vi "Listbox demo.vi"() -> ()   [LabVIEW 2012, in "Queue FIFO.lvlib"]
uses:
  Queue FIFO.lvlib
panel:
  in  "停止":bool
  in  "列表框":i32(listbox)
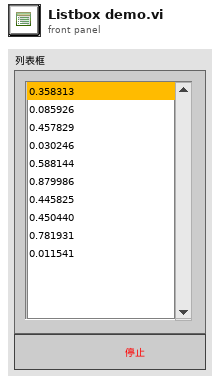
[diagram p1: front panel]
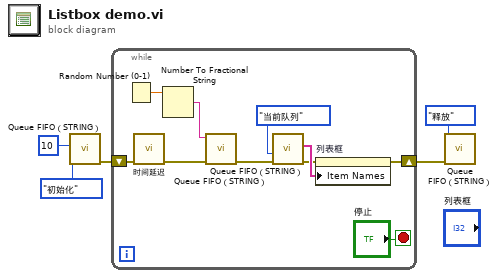
[diagram p0: block diagram]
diagram:
  n1 = call "Queue FIFO（STRING）.vi"("模式"=enum16{"初始化", "加入元素", "当前队列", "释放"}."初始化", "length"=10) -> ("error out"=w3:errorcluster)  [unwired: 6 in, 3 out]
  n2 = while {
    shift-right: [w6] -> w2
    shift-left: w3 -> [w15]
    stop <- "停止" stop-if-true
    n3 = Random Number (0-1)() -> (number: 0 to 1=w13:dbl)
    n4 = call "时间延迟"("error in (no error)"=w15) -> ("error out"=w14:errorcluster)  [unwired: 10 in]
    n5 = Number To Fractional String(number=w13) -> (F-format string=w12:string)  [unwired: 3 in]
    n6 = call "Queue FIFO（STRING）.vi"("error in (no error)"=w14, "输入"=w12) -> ("error out"=w10:errorcluster)  [unwired: 6 in, 3 out]
    n7 = call "Queue FIFO（STRING）.vi"("error in (no error)"=w10, "模式"=enum16{"初始化", "加入元素", "当前队列", "释放"}."当前队列") -> ("error out"=w7:errorcluster, "当前队列"=w8:string[])  [unwired: 6 in, 2 out]
    n8 = property on="列表框" class="LstBox (严格)"(error in=w7, "Item Names"=w8) -> (error out=w6:errorcluster)  [unwired: 1 in, 1 out]
  }
  n9 = call "Queue FIFO（STRING）.vi"("error in (no error)"=w2, "模式"=enum16{"初始化", "加入元素", "当前队列", "释放"}."释放") -> ()  [unwired: 6 in, 4 out]
